vi "MovCor-Generate timestamps sequence.vi"(7 "ROI Dwell time (us)":dbl=4.0 min=0.05 max=20.0 step=0.05, 9 "Time resolution of simulated waveform":dbl, 10 "High value of simulated waveform":dbl, 11 "Acquisition system simulated waveform":waveform(dbl)) -> (1 "Time-stamps (us)":dbl[](array[numeric]) format="%.2f", 3 "Number of timestamp indexes":i32)   [LabVIEW 2020]
uses:
  <userlib>/_OpenG.lib/array/array.llb/Search 1D Array (DBL)__ogtk.vi
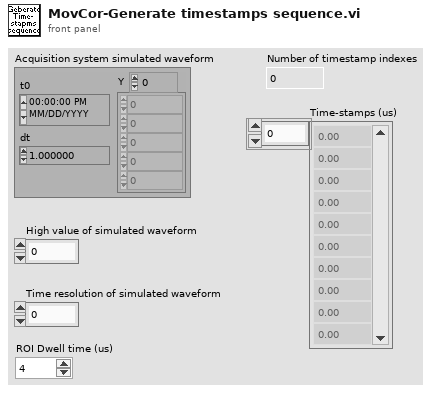
[diagram p1: front panel]
types:
  T1 = typedef "AOL_Globals.ctl" = cluster{"Imaging Protocol":T2, "Number of POI":u16, "Number of Miniscans":u16, "Number of Trials":u16, "Number of Cycles ":u64, "# Averaged Frames":u16, "Laser power (%)":u8, "Pockels (V)":dbl, "Acquisition Length (sec)":dbl, "Fill time (us)":dbl, "POI Dwell time (us)":dbl, "Miniscan Dwell time per pixel (us)":dbl, "PMT 1":dbl, "PMT 2":dbl, "Back Apperture (mA)":dbl, "Frame Size":T3, "Center Frequency":dbl, "Field of View (norm)":dbl, "DwellTime (us)":dbl, "Wavelength (nm)":dbl, "Zoom":dbl, "AOL Z":dbl, "AOL Mode":T4, "GridXY":dbl, "GridZ":dbl, "TriggerPeriod (sec)":dbl, "Number of Pixels in Miniscan":u16, "Experiment folder path":path, "X centre":dbl, "Y centre":dbl, "Angle (degrees)":dbl, "Plane Mode":T5, "Threshold":u16[], "Regenerate Chirps":bool, "Rectangle ROI length (pixels)":u16, "Rectangle ROI height (pixels)":u16, "AOD fill":u16, "StartupDelay":i32, "Samples Wait after Trigger":u16, "Slip Cycle":u32, "Add Cycle":bool, "Functional Mode":T6, "Z Start":dbl, "Z Stop":dbl, "# Planes":i32, "Total Pixels":i32, "Variable Miniscan Pixels":u16[], "Use Variable Length":bool, "Use Variable Resolution":bool, "Laser power (%) at Z Start":u8, "Laser power (%) at Z Stop":u8, "Ref Z Step":i8, "Ref Dwell Time (us)":dbl, "Field of View (um)":dbl}
  T2 = typedef "Imaging Protocols enum.ctl" = enum16{"AOL Z-Stack", "Motor Z Stack", "Functional Acquisition", "Single Plane Acquisition", "Volume Acquisition", "Live Imaging", "Live Plane Imaging", "Live Volume Imaging"}
  T3 = typedef "Frame Size.ctl" = u16
  T4 = typedef "AOL modes.ctl" = enum16{"Raster", "Structural", "Pointing", "Mini Scan", "Alignment"}
  T5 = typedef "Plane Mode.ctl" = u16
  T6 = typedef "Functional Mode.ctl" = enum16{"Point", "Line", "Patch", "Plane", "Volume"}
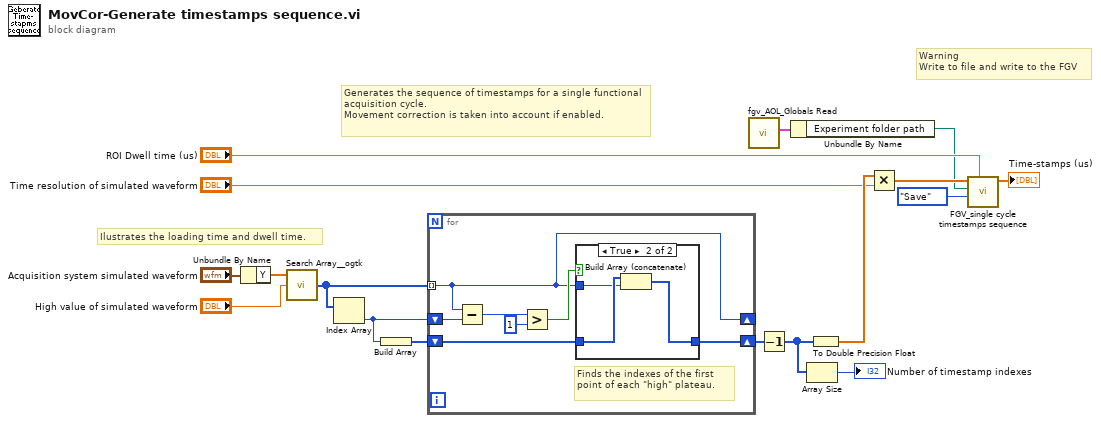
[diagram p0: block diagram]
diagram:
  # "Warning\nWrite to file and write to the FGV"
  # "Generates the sequence of timestamps for a single functional acquisition cycle.\nMovement correction is taken into account if enabled."
  # "Ilustrates the loading time and dwell time."
  n1 = Unbundle By Name ("Get Waveform Components")("Acquisition system simulated waveform") -> ("Y"=w14:dbl[])
  n2 = call-poly <userlib>:"Search Array__ogtk.vi"("Array"=w14, "Element Data"="High value of simulated waveform") -> ("Indices of Elements"=w12:i32[])  [unwired: 7 in]
  n3 = Index Array(array=w12) -> (element=w11:i32)  [unwired: 1 in]
  n4 = Build Array(w11) -> (w10:i32[])
  n5 = for {
    shift-right: [w23] -> w15
    shift-left: w10 -> [w24]
    shift-right: [w18] -> _
    shift-left: w11 -> [w22]
    tunnel: w12 -> [w18] mode=indexing
    # "Finds the indexes of the first point of each \"high\" plateau."
    n6 = Subtract(x=w18, y=w22) -> (x-y=w21:i32)
    n7 = Greater?(x=w21, y=1) -> (0:w19:bool)
    n8 = case shown="True" w19 {
      tunnel: w24 -> [w25 w28]
      tunnel: [w25 w27] -> w23
      tunnel: w18 -> [_ w26]
      frame False {
      }
      frame True {
        n9 = Build Array (concatenate)(w28, w26) -> (w27:i32[])
      }
    }
  }
  n10 = call "fgv_AOL_Globals Read.vi"() -> ("AOL_Globals"=w2:T1)  [unwired: 9 in, 2 out]
  n11 = Decrement(x=w15) -> (x-1=w6:i32[])
  n12 = Unbundle By Name(w2) -> ("Experiment folder path"=w1:path)
  n13 = Array Size(array=w6) -> (size(s)=→"Number of timestamp indexes":i32)
  n14 = To Double Precision Float(number=w6) -> (double precision float=w17:dbl[])
  n15 = Multiply(x=w17, y="Time resolution of simulated waveform") -> (x*y=w7:dbl[])
  n16 = call "FGV_single cycle timestamps sequence.vi"("ROI Dwell time (us)"="ROI Dwell time (us)", "Function"=enum16{"Read", "Write", "Load", "Save"}."Save", "Experiment folder path"=w1, "Time-stamps (us) in"=w7) -> ("Single funct.acq cycle time-stamps (us)"=→"Time-stamps (us)":dbl[])  [unwired: 6 in, 1 out]
